vi "Waveforms.vi"(9 "Digital Data":digitaldata={"transitions"=[3, 7, 8], "data"=[[0, 0, 0, 0, 0, 0, 0, 0, 0, 0], [0, 0, 1, 1, 1, 1, 0, 0, 1, 1], [1, 1, 0, 1, 0, 1, 1, 0, 0, 1]]}, 10 "Digital Waveform":digitalwaveform(waveform)={"t0"=timestamp(3383028711.362774 s since 1904-01-01), "dt"=3.0, "Y"={"transitions"=[11, 17, 23], "data"=[[1, 1, 0, 1, 0, 0, 1, 0, 0, 1, 1, 1, 0, 0], [1, 0, 0, 1, 1, 1, 1, 0, 0, 0, 0, 0, 0, 0], [0, 0, 1, 0, 1, 0, 1, 1, 1, 0, 0, 1, 1, 1]]}}, 11 "Waveform":waveform(dbl)={"t0"=timestamp(3382631016.906947 s since 1904-01-01), "dt"=-2.0, "Y"=[11.0, 209.0]}) -> ()   [LabVIEW 2009]
panel:
  in  "Array":waveform(u32)[](array[waveform])=[{"t0"=timestamp(3383140487.924 s since 1904-01-01), "dt"=2.0, "Y"=[11, 209, 222, 433]}, {"t0"=timestamp(3382631016.906947 s since 1904-01-01), "dt"=-3.0, "Y"=[132, 11]}]
  in  "stop":bool
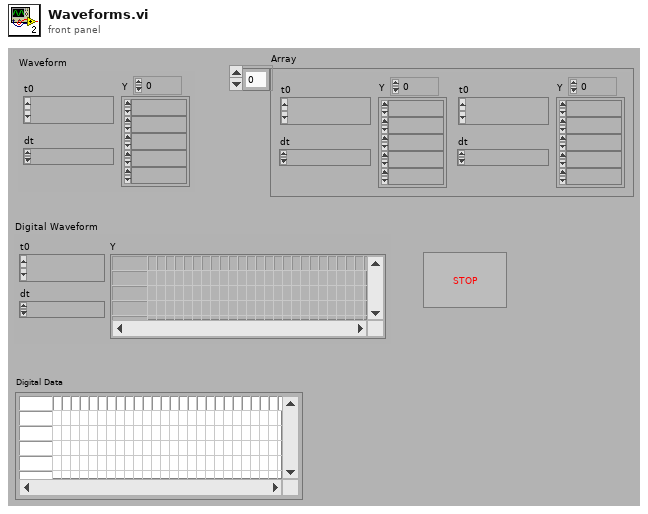
[diagram p1: front panel]
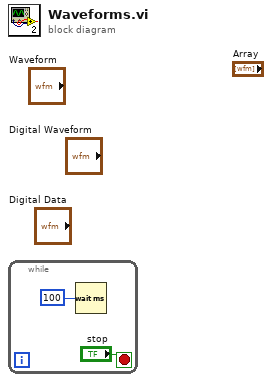
[diagram p0: block diagram]
diagram:
  n1 = while {
    stop <- "stop" stop-if-true
    n2 = Wait (ms)(milliseconds to wait=u32 100) -> ()  [unwired: 1 out]
  }
